vi "Table.vi"(5 "模式":enum16{"select", "insert", "update", "delete"}(ring), 7 "productsName":string, 9 "Table 2":refnum<vi>, 11 "Table":refnum<vi>) -> ()   [LabVIEW 2013]
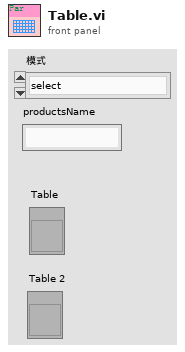
[diagram p1: front panel]
types:
  T1 = enum16{"selectdata", "selectsave", "selectlist", "selectshow"}
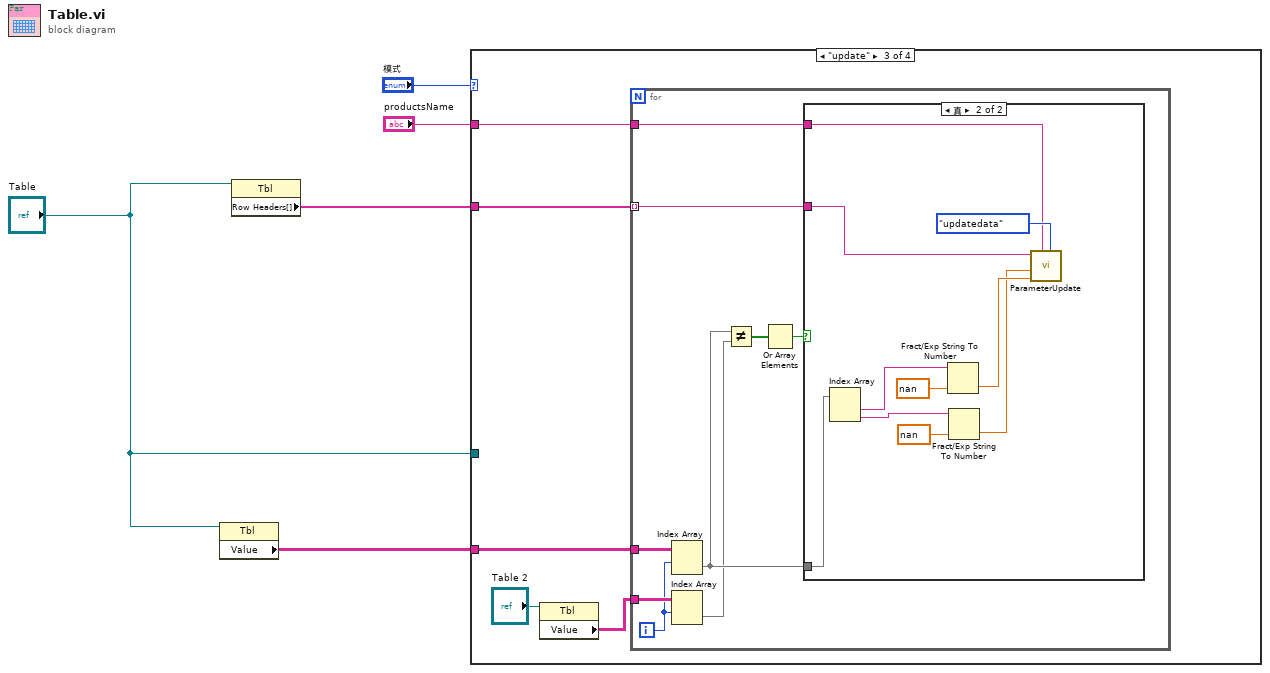
[diagram p0: block diagram]
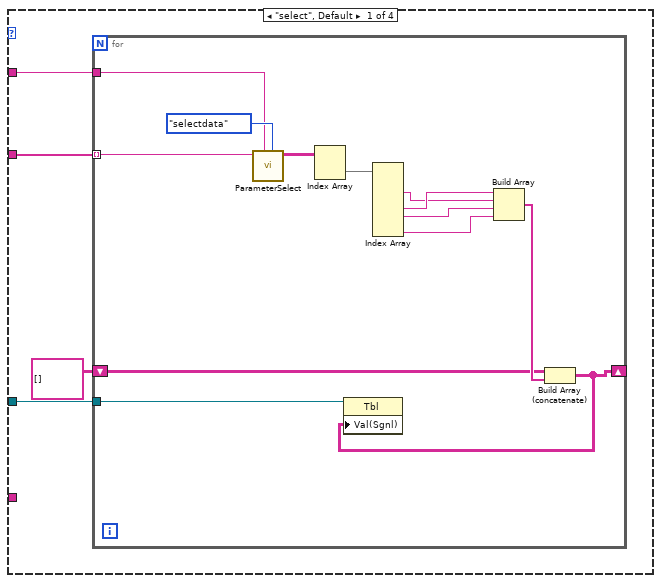
[diagram p2: hidden frame]
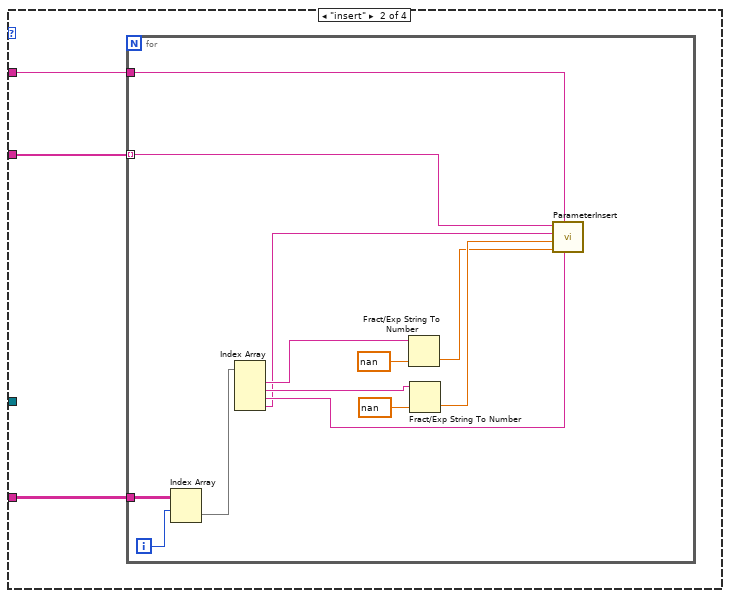
[diagram p3: hidden frame]
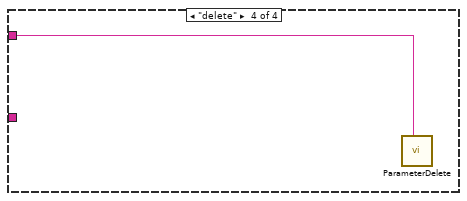
[diagram p5: hidden frame]
diagram:
  n1 = property class="Tbl"(reference="Table") -> ("Value"=w2:string[][])  [unwired: 1 in, 2 out]
  n2 = property class="Tbl"(reference="Table") -> ("Row Headers[]"=w5:string[])  [unwired: 1 in, 2 out]
  n3 = case shown="\"update\"" "模式" {
    tunnel: "productsName" -> [w9 w25 w43 w63]
    tunnel: w5 -> [w8 w24 w42 _]
    tunnel: w2 -> [_ w23 w41 _]
    tunnel: "Table" -> [w7 _ _ _]
    frame "select", Default {
      n4 = for {
        tunnel: w9 -> [w20]
        tunnel: w8 -> [w19] mode=indexing
        shift-right: [w11] -> _
        shift-left: string[][] [] -> [w12]
        tunnel: w7 -> [w13]
        n5 = call "ParameterSelect.vi"("模式"=T1."selectdata", "productsName"=w20, "parameterName"=w19) -> ("dataOutAll"=w22:string[][])  [unwired: 3 in, 5 out]
        n6 = Index Array(array=w22) -> (element=w18:string[])  [unwired: 2 in]
        n7 = Index Array(array=w18) -> (element #2=w15:string, element #4=w16:string, element #5=w17:string, element #7=w10:string)  [unwired: 7 in, 3 out]
        n8 = Build Array(w16, w15, w17, w10) -> (w14:string[])
        n9 = Build Array (concatenate)(w12, w14) -> (w11:string[][])
        n10 = property class="Tbl"(reference=w13, "Val(Sgnl)"=w11) -> ()  [unwired: 1 in, 2 out]
      }
    }
    frame "insert" {
      n11 = for {
        tunnel: w25 -> [w33]
        tunnel: w24 -> [w32] mode=indexing
        tunnel: w23 -> [w31]
        i -> [w30]
        n12 = Index Array(array=w31, index (row)=w30) -> (element=w29:string[])  [unwired: 1 in]
        n13 = Index Array(array=w29) -> (element #1=w37:string, element #2=w35:string, element #3=w34:string, element #4=w26:string)  [unwired: 4 in]
        n14 = Fract/Exp String To Number(string=w37, default (0 dbl)=nan ("默认(0 DBL)")) -> (number=w27:dbl)  [unwired: 2 in, 1 out]
        n15 = Fract/Exp String To Number(string=w35, default (0 dbl)=nan ("默认(0 DBL)")) -> (number=w28:dbl)  [unwired: 2 in, 1 out]
        n16 = call "ParameterInsert.vi"("unit"=w34, "productsName"=w33, "limitL"=w27, "limitH"=w28, "notes"=w26, "parameterName"=w32) -> ()  [unwired: 6 in]
      }
    }
    frame "update" {
      n17 = property class="Tbl"(reference="Table 2") -> ("Value"=w39:string[][])  [unwired: 1 in, 2 out]
      n18 = for {
        tunnel: w43 -> [w52]
        tunnel: w42 -> [w51] mode=indexing
        tunnel: w41 -> [w50]
        tunnel: w39 -> [w49]
        i -> [w48]
        n19 = Index Array(array=w50, index (row)=w48) -> (element=w47:string[])  [unwired: 1 in]
        n20 = Index Array(array=w49, index (row)=w48) -> (element=w46:string[])  [unwired: 1 in]
        n21 = Not Equal?(x=w47, y=w46) -> (x != y?=w45:bool[])
        n22 = Or Array Elements ("数组元素或操作")(Boolean array=w45) -> (logical OR=w44:bool)
        n23 = case shown="真" w44 {
          tunnel: w52 -> [_ w59]
          tunnel: w51 -> [_ w58]
          tunnel: w47 -> [_ w53]
          frame False {
          }
          frame True {
            n24 = Index Array(array=w53) -> (element #1=w57:string, element #2=w56:string)  [unwired: 2 in]
            n25 = Fract/Exp String To Number(string=w57, default (0 dbl)=nan ("默认(0 DBL)")) -> (number=w55:dbl)  [unwired: 2 in, 1 out]
            n26 = Fract/Exp String To Number(string=w56, default (0 dbl)=nan ("默认(0 DBL)")) -> (number=w54:dbl)  [unwired: 2 in, 1 out]
            n27 = call "ParameterUpdate.vi"("模式"=enum16{"updatedata", "updatesave"}."updatedata", "productsName"=w59, "limitL"=w55, "limitH"=w54, "parameterName"=w58) -> ()  [unwired: 7 in]
          }
        }
      }
    }
    frame "delete" {
      n28 = call "ParameterDelete.vi"("productsName"=w63) -> ()  [unwired: 11 in]
    }
  }
